vi "Write SGL as Numeric.vi"(8 "error in (no error)":errorcluster, 9 "Numeric":sgl, 10 "Tag":string, 11 "Omni_Bus in":refnum<class "Omni_Bus.lvclass">) -> (0 "error out":errorcluster, 3 "Omni_Bus out":refnum<class "Omni_Bus.lvclass">)   [LabVIEW 2021, in "Omni_Bus.lvclass"]
uses:
  Omni_Bus.lvclass
  Omni_Bus.lvclass/Omni_Bus.ctl
  <vilib>/TSA/Abstract Data Classes/Abs_Types/Numeric/Abs_Numeric.lvclass
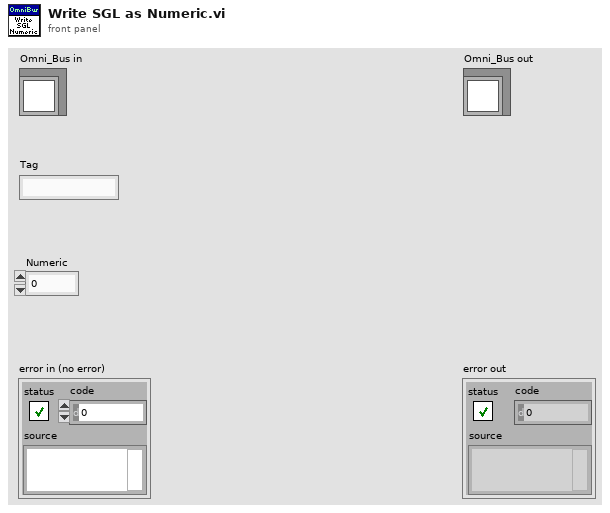
[diagram p1: front panel]
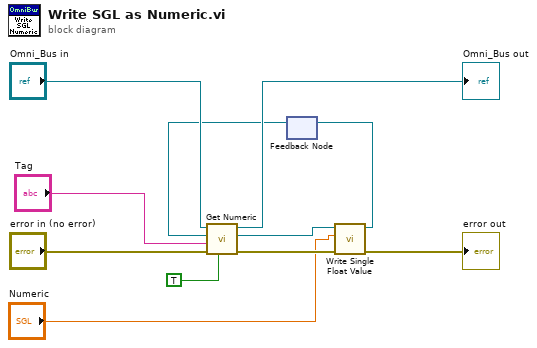
[diagram p0: block diagram]
diagram:
  n1 = feedback #1() -> (w3:refnum<class "Abs_Numeric.lvclass">)  [unwired: 1 in]
  n2 = call-dynamic "Get Numeric.vi"("Write?"=TRUE, "error in (no error)"="error in (no error)", "Tag"="Tag", "Value Type"=w3, "Var Bus in"="Omni_Bus in") -> ("error out"=w7:errorcluster, "Value Out"=w4:refnum<class "Abs_Numeric.lvclass">, "Var Bus out"=→"Omni_Bus out":refnum<class "Omni_Bus.lvclass">)  [unwired: 4 in]
  n3 = call-dynamic "Write Single Float Value.vi"("error in (no error)"=w7, "Float"="Numeric", "Numeric in"=w4) -> ("error out"=→"error out":errorcluster, "Numeric out"=w5:refnum<class "Abs_Numeric.lvclass">)  [unwired: 7 in]
  n4 = feedback-in #1(w5) -> ()
